vi "Clear Macro Sections.vi"(8 "error in (no error)":errorcluster, 11 "refnum":T1) -> (0 "error out":errorcluster, 3 "refnum out":T1)   [LabVIEW 2020, in "MacroAssert.lvlib"]
doc: "Clears all sections from the macro config file defined by <B>refnum</B>."
uses:
  MacroAssert.lvlib
  <vilib>/Utility/config.llb/Config Data RefNum.ctl
  <vilib>/Utility/config.llb/NI_LVConfig.lvlib
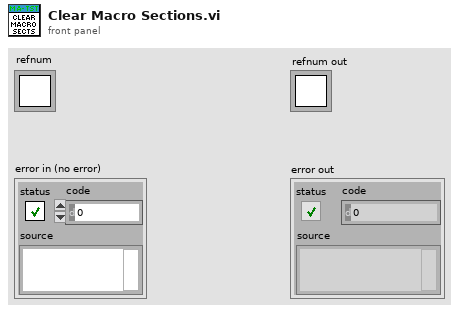
[diagram p1: front panel]
types:
  T1 = typedef "NI_LVConfig.lvlib/Config Data RefNum.ctl" = refnum<k1>
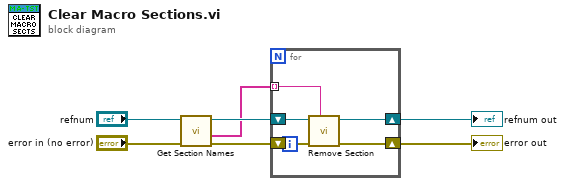
[diagram p0: block diagram]
diagram:
  n1 = call <vilib>:"Get Section Names.vi"("error in (no error)"="error in (no error)", "refnum"="refnum") -> ("error out"=w5:errorcluster, "section names"=w3:string[], "refnum out"=w4:T1)  [unwired: 7 in]
  n2 = for {
    shift-right: [w8] -> w1
    shift-left: w5 -> [w11]
    shift-right: [w9] -> w2
    shift-left: w4 -> [w12]
    tunnel: w3 -> [w10] mode=indexing
    n3 = call <vilib>:"Remove Section.vi"("section"=w10, "error in (no error)"=w11, "refnum"=w12) -> ("error out"=w8:errorcluster, "refnum out"=w9:T1)  [unwired: 6 in, 1 out]
  }
  "error out" <- w1
  "refnum out" <- w2
